vi "StringArray2CharBuffer.vi"(1 "elementDescription":string[](array[string])) -> (0 "Array":u8[](array[numeric]))   [LabVIEW 2009]
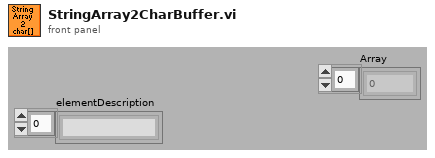
[diagram p1: front panel]
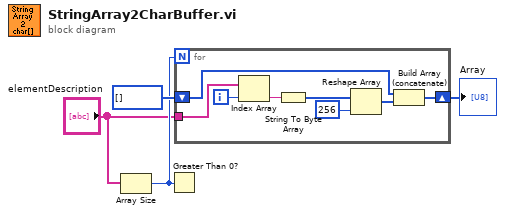
[diagram p0: block diagram]
diagram:
  n1 = Array Size(array="elementDescription") -> (size(s)=w3:i32)
  n2 = Greater Than 0?(x=w3) -> ()  [unwired: 1 out]
  n3 = for {
    N: w3 -> [_]
    tunnel: "elementDescription" -> [w12]
    shift-right: [w5] -> w1
    shift-left: u8[] [] ("Array") -> [w6]
    i -> [w10]
    n4 = Index Array(array=w12, index=w10) -> (element=w11:string)
    n5 = String To Byte Array(string=w11) -> (unsigned byte array=w9:u8[])
    n6 = Reshape Array(w9, 256 ("dimension size")) -> (w7:u8[])
    n7 = Build Array (concatenate)(w6, w7) -> (w5:u8[])
  }
  "Array" <- w1
